vi "SSC Digital Read Sequencer Register.vi"(0 "Digital SSC in":T1[](array[typedef]), 5 "Sequencer Register":string(combo)="reg0", 11 "error in":errorcluster) -> (4 "Digital SSC out":T1[](array[typedef]), 6 "Per-Instrument Register Values":i32[](array[numeric]), 15 "error out":errorcluster)   [LabVIEW 2020]
doc: "Reads the value of a pattern sequencer register on the device(s) connected to the specified pin(s) and pin group(s). Use pattern sequencer registers to pass numeric values between the pattern sequencer and a runtime test program."
uses:
  SSC Digital.ctl
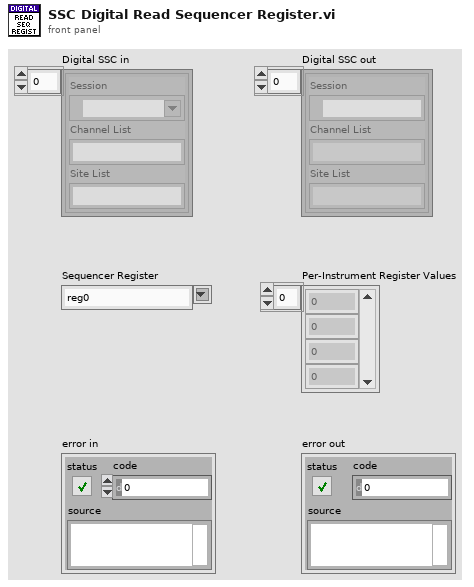
[diagram p1: front panel]
types:
  T1 = typedef "SSC Digital.ctl" = cluster{"Session":refnum<k15>, "Channel List":string, "Site List":string}
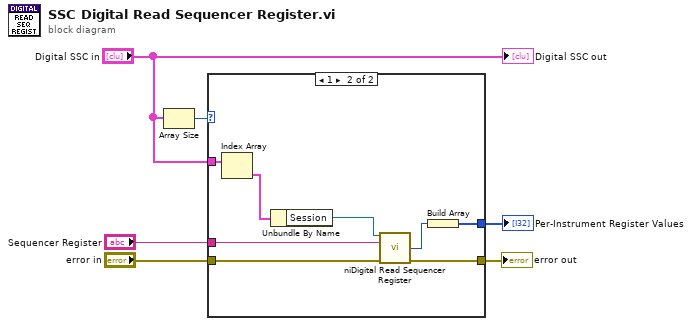
[diagram p0: block diagram]
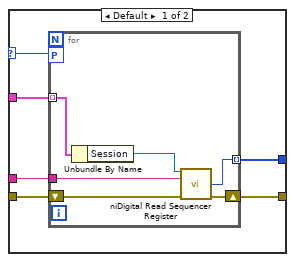
[diagram p2: hidden frame]
diagram:
  n1 = Array Size(array="Digital SSC in") -> (size(s)=w2:i32)
  n2 = case shown="1" w2 {
    selector: w2 -> [w8 _]
    tunnel: [w12 w26] -> w6
    tunnel: "error in" -> [w11 w25]
    tunnel: [w10 w19] -> w4
    tunnel: "Sequencer Register" -> [w9 w23]
    tunnel: "Digital SSC in" -> [w7 w22]
    frame Default {
      n3 = for {
        tunnel: w7 -> [w18] mode=indexing
        workers-P: w8 -> [_]
        tunnel: [w14] -> w10 mode=indexing
        tunnel: w9 -> [w13]
        shift-right: [w16] -> w12
        shift-left: w11 -> [w17]
        n4 = Unbundle By Name(w18) -> ("Session"=w15:refnum<k15>)
        n5 = call <instrlib>:"niDigital Read Sequencer Register.vi"("instrument handle"=w15, "sequencer register"=w13, "error in"=w17) -> ("value"=w14:i32, "error out"=w16:errorcluster)  [unwired: 10 in, 1 out]
      }
    }
    frame 1 {
      n6 = Index Array(array=w22) -> (element=w20:T1)  [unwired: 1 in]
      n7 = Unbundle By Name(w20) -> ("Session"=w21:refnum<k15>)
      n8 = call <instrlib>:"niDigital Read Sequencer Register.vi"("instrument handle"=w21, "sequencer register"=w23, "error in"=w25) -> ("value"=w24:i32, "error out"=w26:errorcluster)  [unwired: 10 in, 1 out]
      n9 = Build Array(w24) -> (w19:i32[])
    }
  }
  "error out" <- w6
  "Per-Instrument Register Values" <- w4
  "Digital SSC out" <- "Digital SSC in"
